vi "Wrap Value.vi"(10 "Max":i32, 11 "Value":i32) -> (3 "Value Wrapped":i32)   [LabVIEW 2021, in "Camera.lvclass"]
uses:
  Camera.lvclass
  Camera.lvclass/Camera.ctl
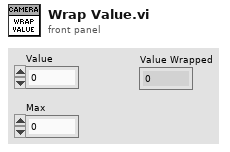
[diagram p1: front panel]
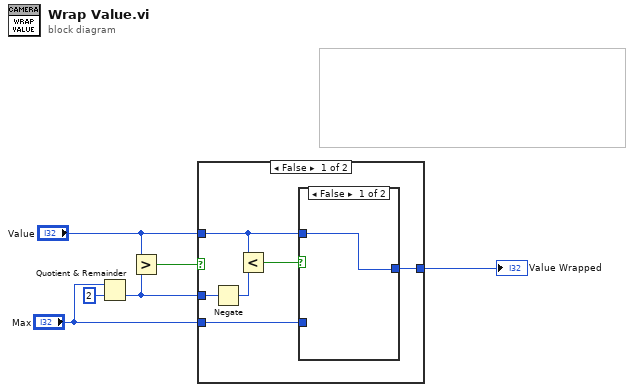
[diagram p0: block diagram]
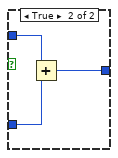
[diagram p2: hidden frame]
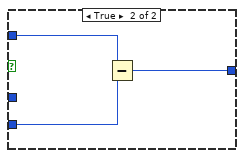
[diagram p3: hidden frame]
diagram:
  n1 = Quotient & Remainder(x="Max", y=2) -> (floor(x/y)=w1:i32)  [unwired: 1 out]
  n2 = Greater?(x="Value", y=w1) -> (0:w6:bool)
  n3 = case shown="False" w6 {
    tunnel: "Value" -> [w9 w19]
    tunnel: "Max" -> [w8 w18]
    tunnel: [w7 w17] -> w2
    tunnel: w1 -> [w12 _]
    frame False {
      n4 = Negate(x=w12) -> (-x=w11:i32)
      n5 = Less?(x=w9, y=w11) -> (x < y?=w10:bool)
      n6 = case shown="False" w10 {
        tunnel: w9 -> [w13 w16]
        tunnel: w8 -> [_ w15]
        tunnel: [w13 w14] -> w7
        frame False {
        }
        frame True {
          n7 = Add(x=w16, y=w15) -> (x+y=w14:i32)
        }
      }
    }
    frame True {
      n8 = Subtract(x=w19, y=w18) -> (x-y=w17:i32)
    }
  }
  "Value Wrapped" <- w2
